vi "Wait for empty queue.vi"(8 "error in (no error)":errorcluster, 9 "timeout":i32=-1, 11 "Queue in":refnum<queue>) -> (0 "error out":errorcluster, 3 "Queue out":refnum<queue>)   [LabVIEW 2013]
uses:
  Data.ctl
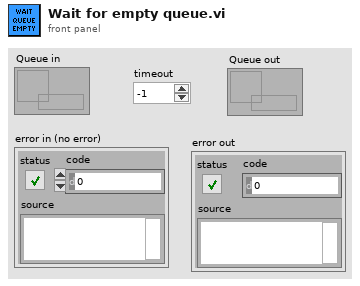
[diagram p1: front panel]
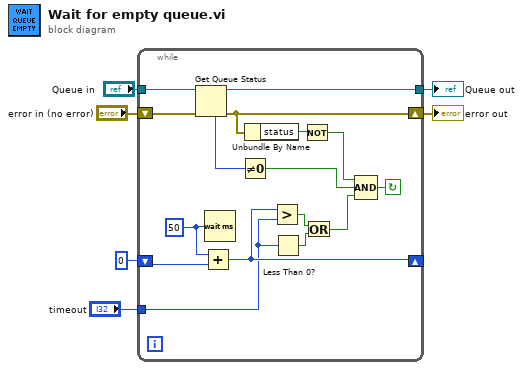
[diagram p0: block diagram]
diagram:
  n1 = while {
    tunnel: "Queue in" -> [w22]
    tunnel: [w20] -> w2
    shift-right: [w16] -> _
    shift-left: 0 -> [w17]
    tunnel: "timeout" -> [w15]
    shift-right: [w9] -> w1
    shift-left: "error in (no error)" -> [w21]
    stop <- w12 continue-if-true
    w18 = u32 50 ("milliseconds to wait")
    n2 = Get Queue Status(queue=w22, error in (no error)=w21) -> (queue out=w20:refnum<queue>, error out=w9:errorcluster, # elements in queue=w19:i32)  [unwired: 1 in, 5 out]
    n3 = Add(x=w18, y=w17) -> (x+y=w16:u32)
    n4 = Wait (ms)(milliseconds to wait=w18) -> ()  [unwired: 1 out]
    n5 = Not Equal To 0?(x=w19) -> (x != 0?=w10:bool)
    n6 = Unbundle By Name(w9) -> ("status"=w8:bool)
    n7 = Greater?(x=w16, y=w15) -> (0:w13:bool)
    n8 = Less Than 0?(x=w15) -> (x < 0?=w14:bool)
    n9 = Not(x=w8) -> (.not. x?=w7:bool)
    n10 = Or(x=w13, y=w14) -> (x .or. y?=w11:bool)
    n11 = Compound Arithmetic op=AND(w7, w10, w11) -> (w12:bool)
  }
  "Queue out" <- w2
  "error out" <- w1
